vi "adc_avg_oversampling.vi"(0 "CCS":T1={"Port Number"=1444, "Core Number"=1, "Page"=0}, 11 "error in":errorcluster) -> (4 "CCS out":T1={"Port Number"=1444, "Core Number"=1, "Page"=0})   [LabVIEW 2019]
uses:
  <userlib>/_TI-LA/Reusable/CCS/APIs/Data/Polymorphics/Write Data To Symbol - U16.vi
  <userlib>/_TI-LA/Reusable/CCS/APIs/Data/Polymorphics/Read Data From Symbol - U16 Array.vi
  <vilib>/Utility/file.llb/Write Delimited Spreadsheet (I64).vi
  <vilib>/Utility/file.llb/Write Delimited Spreadsheet (DBL).vi
  <userlib>/_TI-LA/Reusable/CCS/APIs/CCS.lvlib
panel:
  out "Array 2":dbl[](array[numeric])
  out "size(s)":i32
  out "Array":i32[](array[numeric])
  out "error out":errorcluster
  # "uint16_t lv_ref_sel     =   0; //0=vdda, 1=extref, 2=intref\nuint16_t lv_ref_vol     =   0; //0=2P5V, 1=1P4V\nuint16_t lv_scomp       =   8; //8Clocks of 32M give = 250ns"
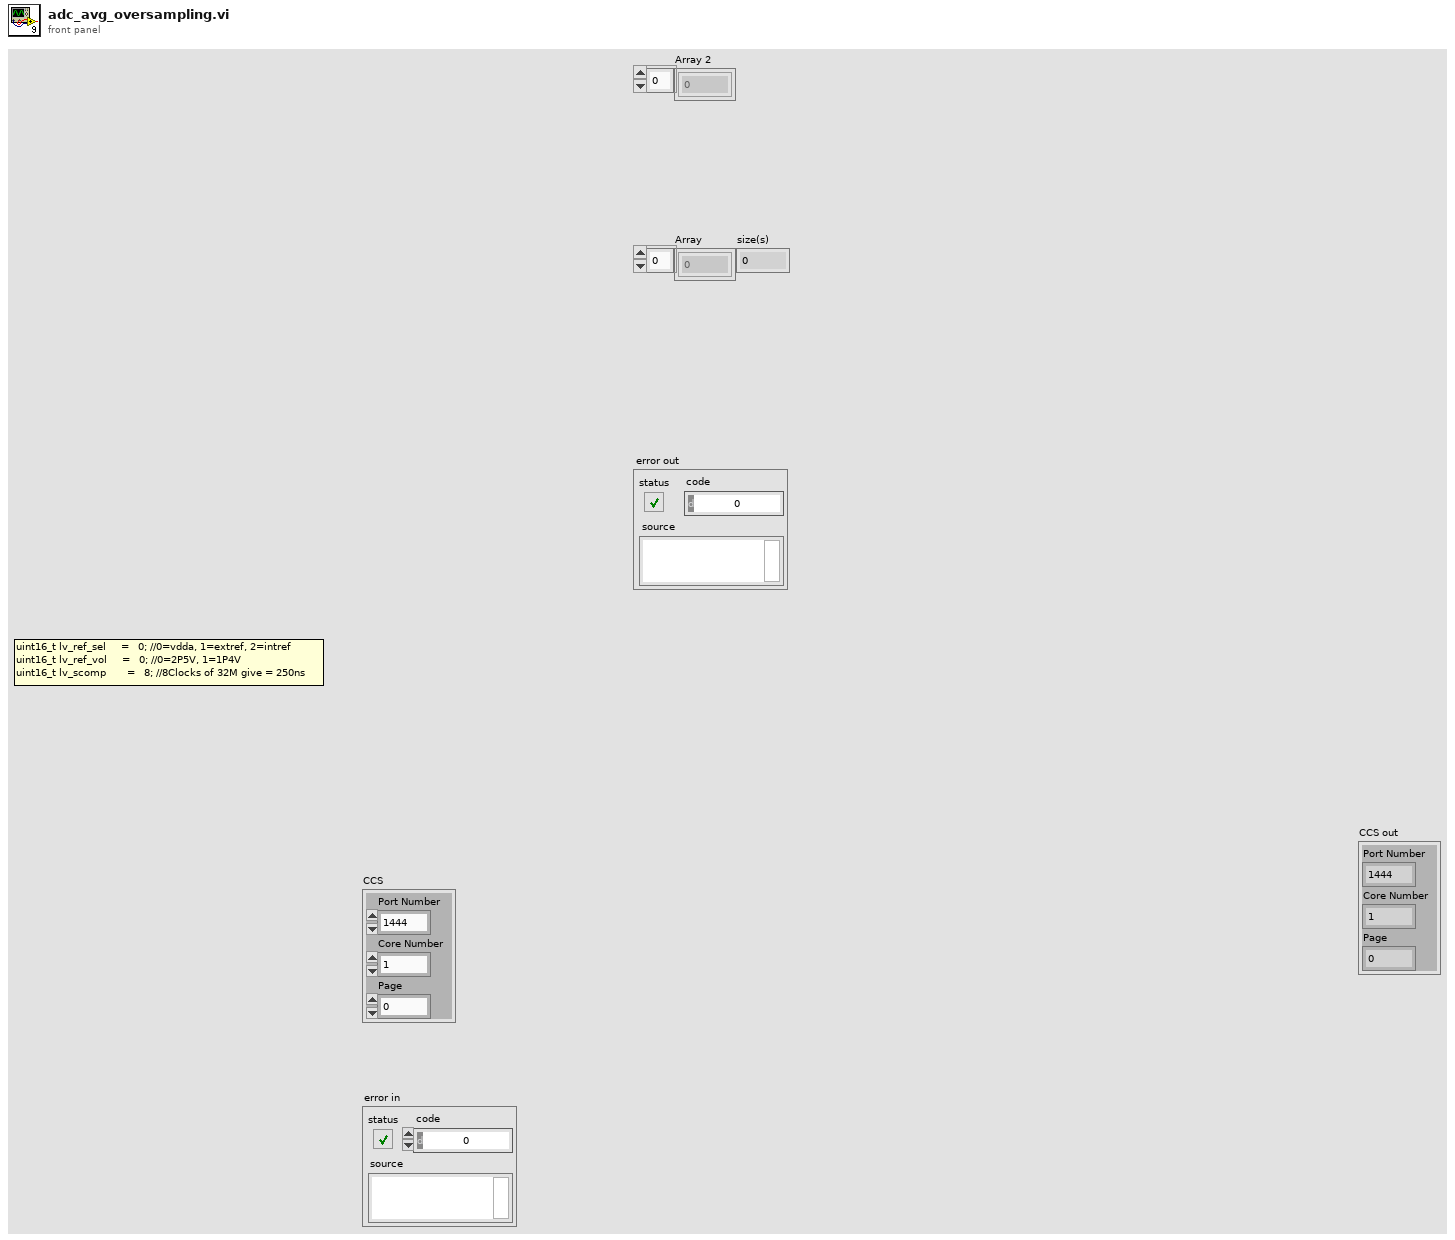
[diagram p1: front panel]
types:
  T1 = cluster{"Port Number":u16, "Core Number":u16, "Page":i32}
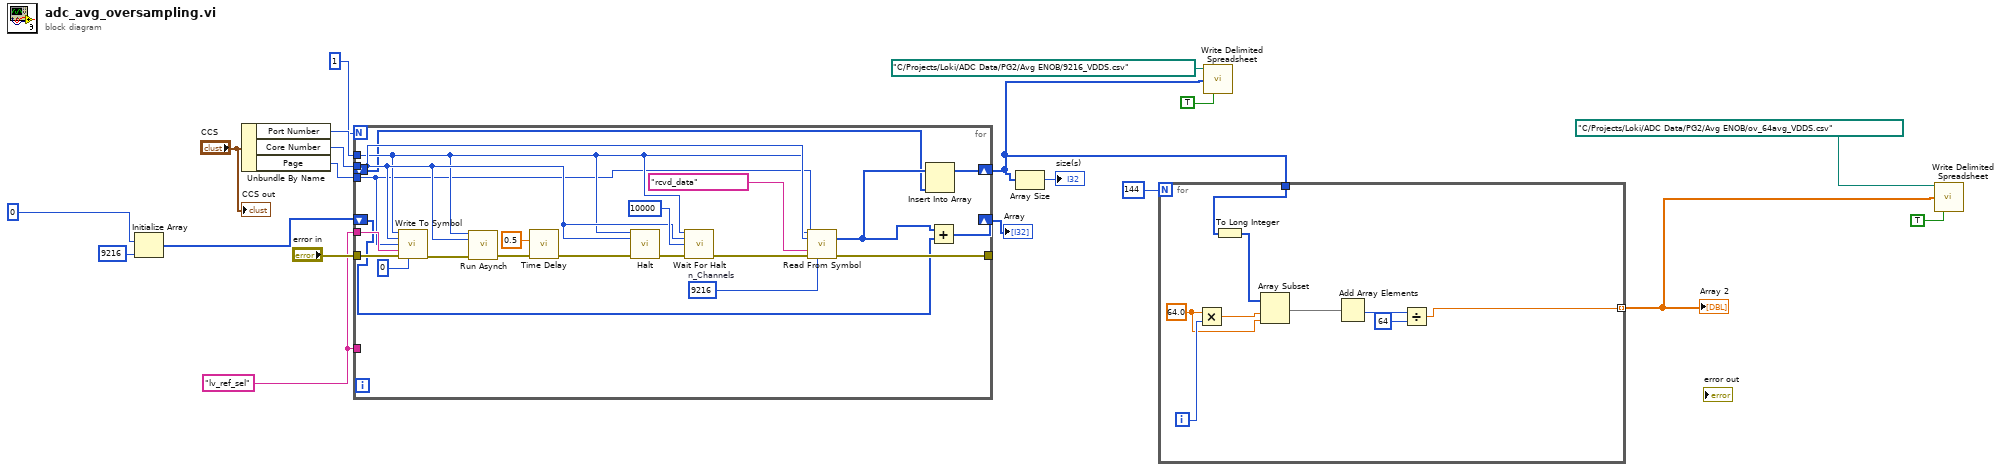
[diagram p0: block diagram]
diagram:
  w13 = "lv_ref_sel"
  n1 = Initialize Array(0, 9216 ("dimension size")) -> (w9:i32[])
  n2 = Unbundle By Name("CCS") -> ("Port Number"=w17:u16, "Core Number"=w15:u16, "Page"=w16:i32)
  n3 = for {
    N: 1 -> [_]
    tunnel: "error in" -> [w35]
    tunnel: w17 -> [w27]
    tunnel: w16 -> [w26]
    tunnel: w15 -> [w28]
    tunnel: w13 -> [w36]
    tunnel: w13 -> [_]
    tunnel: [w25] -> _
    shift-right: [w24] -> w10
    shift-left: w9 -> [w22]
    shift-right: [w21] -> w5
    shift-left: _ -> [w20]
    w40 = u32 9216  # n_Channels
    n4 = call-poly <userlib>:"Write To Symbol.vi"("Port Number"=w27, "Core Number"=w28, "Page"=w26, "Symbol Name"=w36, "error in"=w35, "Write Data"=u16 0) -> ("error out"=w34:errorcluster)  [unwired: 7 in, 2 out]
    n5 = call <userlib>:"Run Asynch.vi"("Port Number"=w27, "Core Number"=w28, "error in"=w34) -> ("error out"=w33:errorcluster)  [unwired: 10 in, 2 out]
    n6 = call "Time Delay"("error in (no error)"=w33, "Delay Time (s)"=0.5) -> ("error out"=w32:errorcluster)  [unwired: 9 in]
    n7 = call <userlib>:"Halt.vi"("Port Number"=w27, "Core Number"=w28, "error in"=w32) -> ("error out"=w38:errorcluster)  [unwired: 10 in, 2 out]
    n8 = call <userlib>:"Wait For Halt.vi"("Port Number"=w27, "Core Number"=w28, "Timeout (10k)(ms)"=10000, "error in"=w38) -> ("error out"=w29:errorcluster)  [unwired: 9 in, 2 out]
    n9 = call-poly <userlib>:"Read From Symbol.vi"("Port Number"=w27, "Core Number"=w28, "Page"=w26, "Symbol Name"="rcvd_data", "error in"=w29, "Data Length"=w40) -> ("Read Data[]"=w23:u16[], "error out"=w25:errorcluster)  [unwired: 6 in, 2 out]
    n10 = Insert Into Array(array=w23, new element=w20) -> (w21:u16[])  [unwired: 1 in]
    n11 = Add(x=w23, y=w22) -> (x+y=w24:i32[])
  }
  "Array" <- w10
  n12 = Array Size(array=w5) -> (size(s)=→"size(s)":i32)
  n13 = for {
    N: 144 -> [_]
    tunnel: w5 -> [w42]
    tunnel: [w43] -> w1 mode=indexing
    i -> [w49]
    w47 = 64.0 ("x")
    n14 = Multiply(x=w47, y=w49) -> (x*y=w48:dbl)
    n15 = To Long Integer(number=w42) -> (32bit integer=w41:i32[])
    n16 = Array Subset(array=w41, index=w48, length=w47) -> (w46:i32[])
    n17 = Add Array Elements(numeric array=w46) -> (sum=w45:i32)
    n18 = Divide(x=w45, y=u16 64) -> (x/y=w43:dbl)
  }
  "Array 2" <- w1
  n19 = call-poly <vilib>:"Write Delimited Spreadsheet.vi"("file path (dialog if empty)"=path "C:/Projects/Loki/ADC Data/PG2/Avg ENOB/9216_VDDS.csv", "1D data"=w5, "transpose? (no:F)"=TRUE) -> ()  [unwired: 11 in, 2 out]
  n20 = call-poly <vilib>:"Write Delimited Spreadsheet.vi"("file path (dialog if empty)"=path "C:/Projects/Loki/ADC Data/PG2/Avg ENOB/ov_64avg_VDDS.csv", "1D data"=w1, "transpose? (no:F)"=TRUE) -> ()  [unwired: 11 in, 2 out]
  "CCS out" <- "CCS"
